vi "Inspect VI.vi"(7 "Inspector Config":T1, 8 "error in (no error)":errorcluster, 11 "VI Path":path=path "C:/dev/SoL/sol-word-search/Scorer (2024Q1)/Scorer/Naughty VI Test.vi") -> (0 "error out":errorcluster, 2 "Issues":string[](array[string]), 3 "Result":bool)   [LabVIEW 2020, in "SoL Inspector.lvlib"]
uses:
  SoL Inspector.lvlib
  Inspector Config.ctl
  Inspection.ctl
  <vilib>/Utility/traverseref.llb/TRef TravTarget.ctl
  <vilib>/Utility/traverseref.llb/VI Scripting - Traverse.lvlib
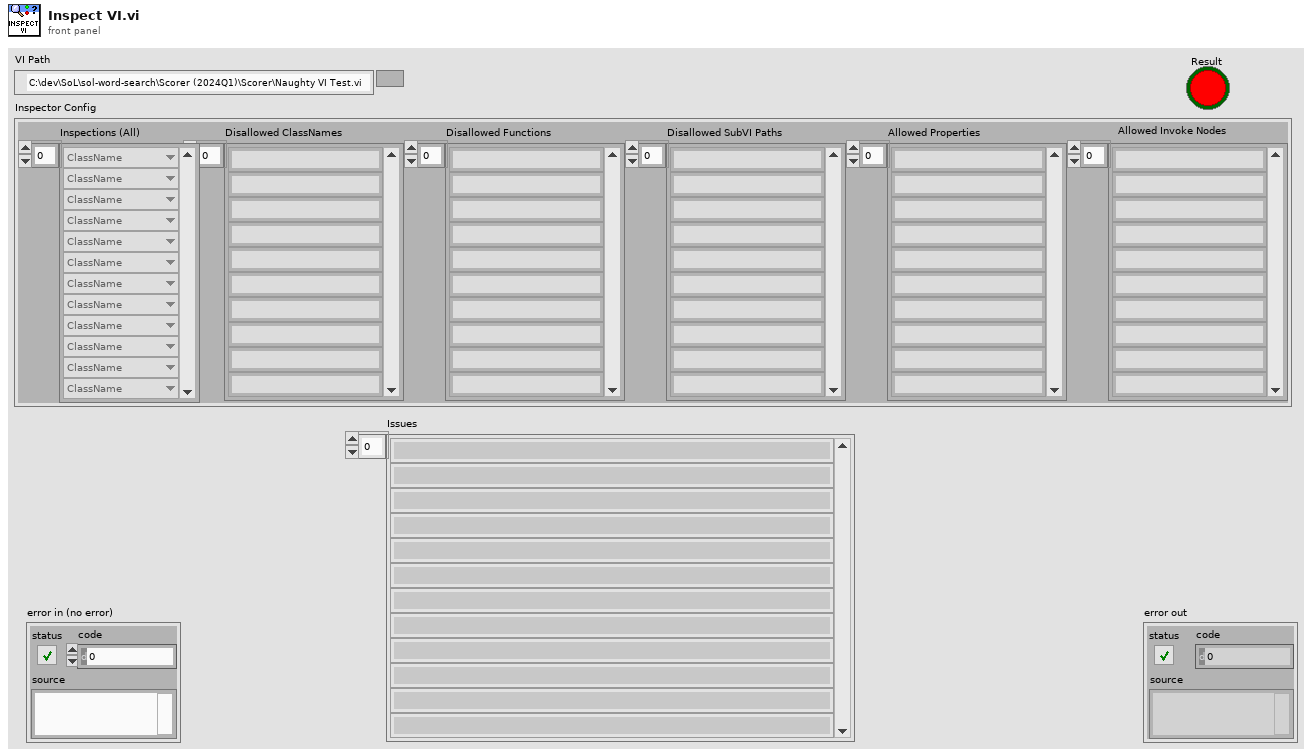
[diagram p1: front panel]
types:
  T1 = typedef "SoL Inspector.lvlib/Inspector Config.ctl" = cluster{"Inspections (All)":T2[], "Disallowed ClassNames":string[], "Disallowed Functions":string[], "Disallowed SubVI Paths":string[], "Allowed Properties":string[], "Allowed Invoke Nodes":string[]}
  T2 = typedef "SoL Inspector.lvlib/Inspection.ctl" = enum16{"ClassName", "Functions", "CallLibrary", "SubVIs", "FileIO", "Invoke Nodes", "Properties", "Growable Functions"}
  T3 = typedef "TRef TravTarget.ctl" = enum16{"FP", "BD", "Other"}
  T4 = typedef "ASPM_UniqueIDStringDatanameShortnameLongname.ctl" = cluster{"Unique ID string":string, "Data name":string, "Short name (localized)":string, "Long name (localized)":string}
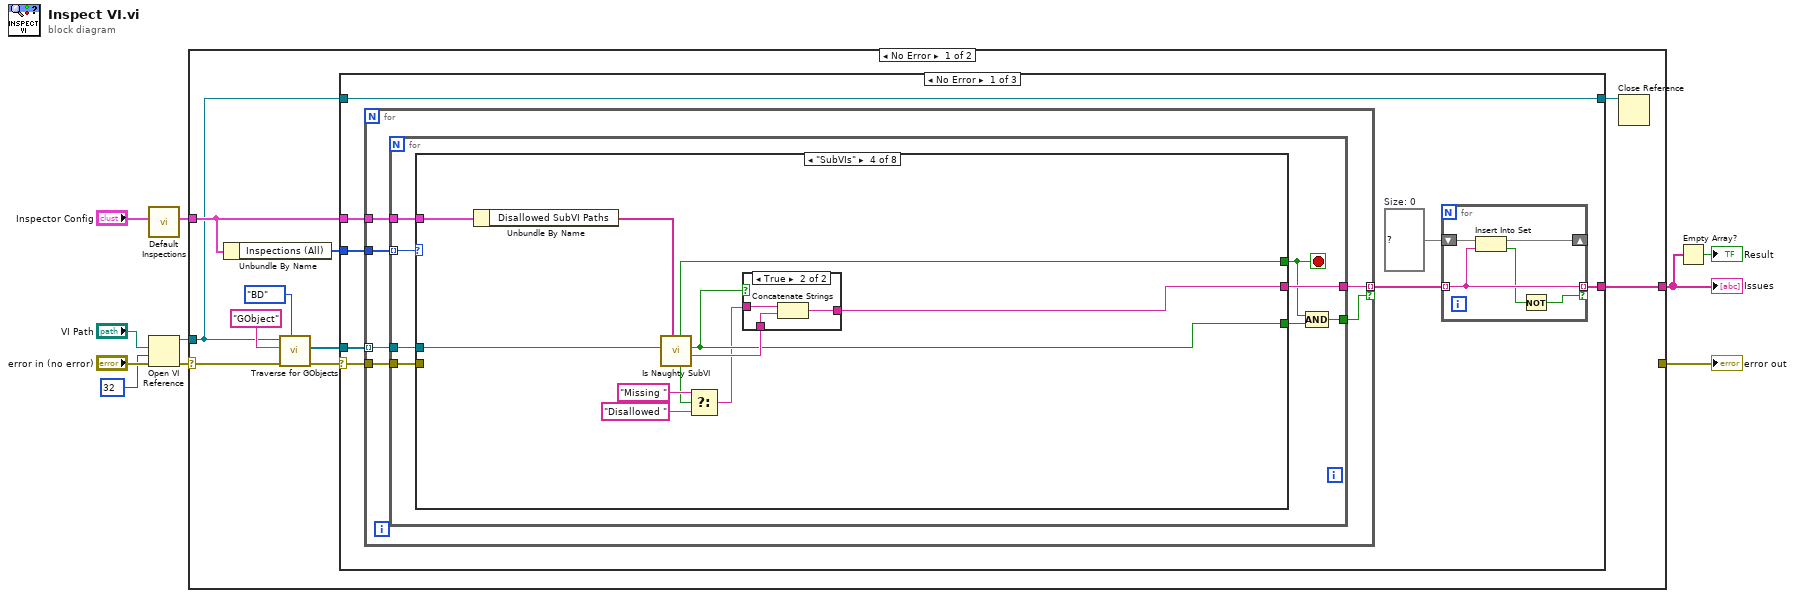
[diagram p0: block diagram]
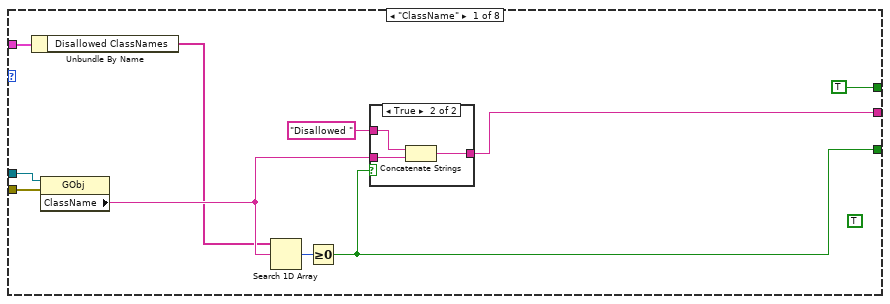
[diagram p2: hidden frame]
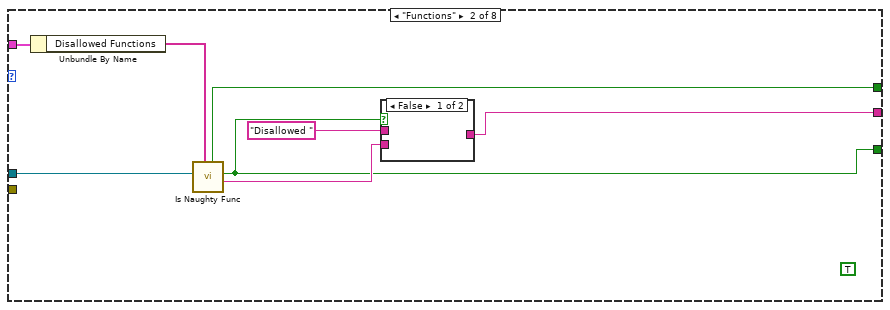
[diagram p4: hidden frame]
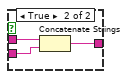
[diagram p5: hidden frame]
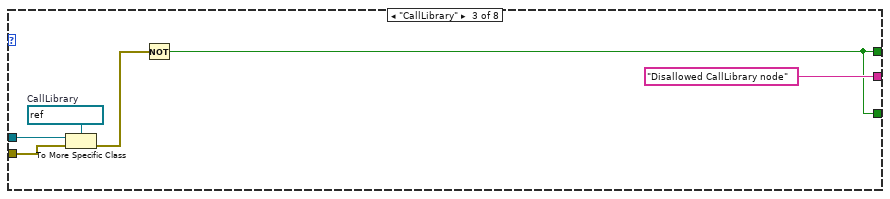
[diagram p6: hidden frame]
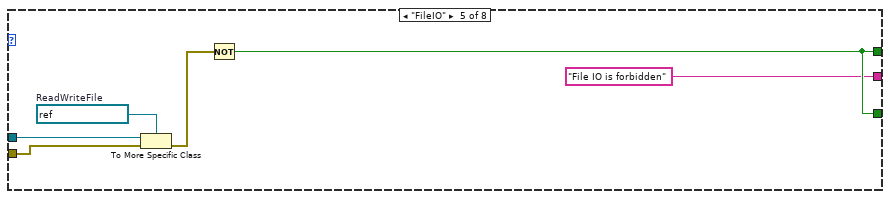
[diagram p8: hidden frame]
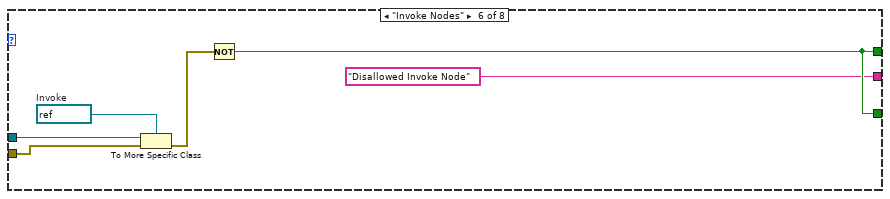
[diagram p9: hidden frame]
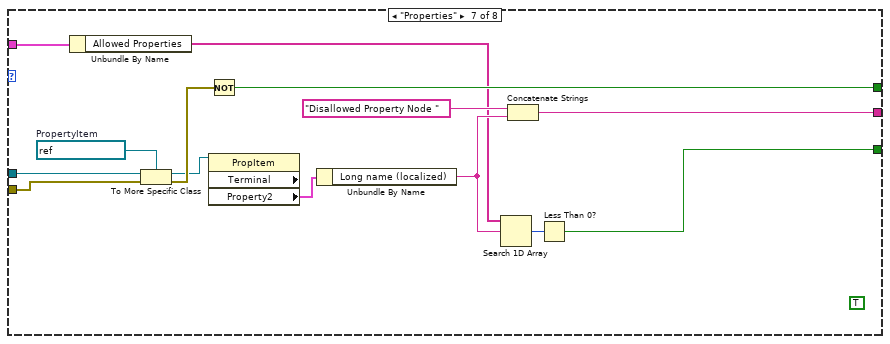
[diagram p10: hidden frame]
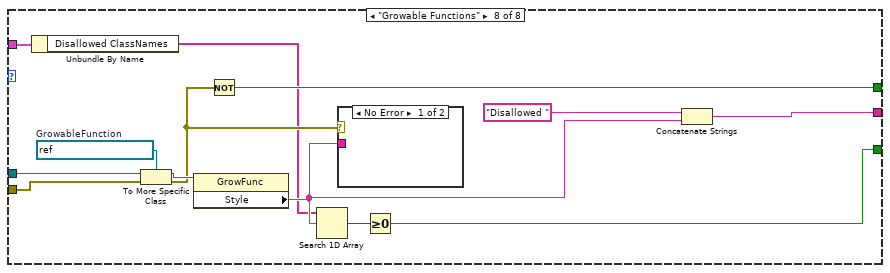
[diagram p11: hidden frame]
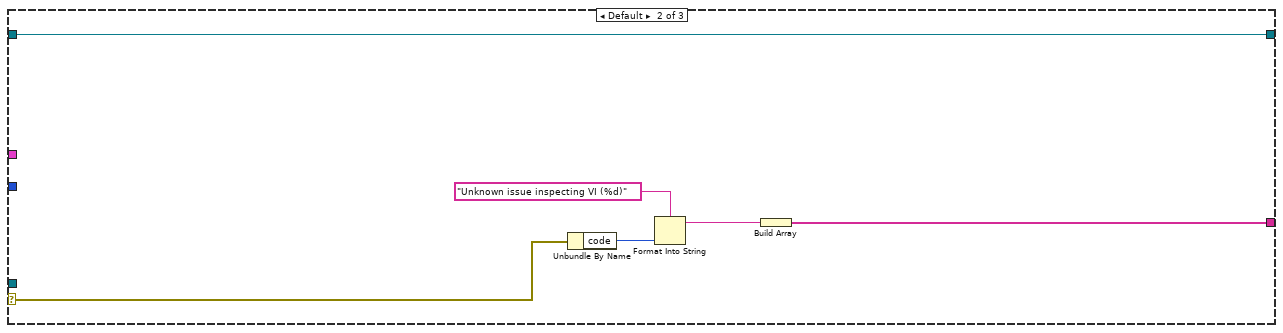
[diagram p13: hidden frame]
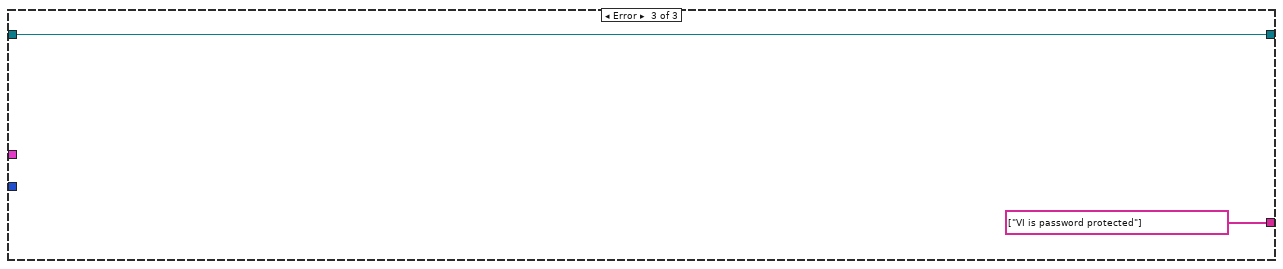
[diagram p14: hidden frame]
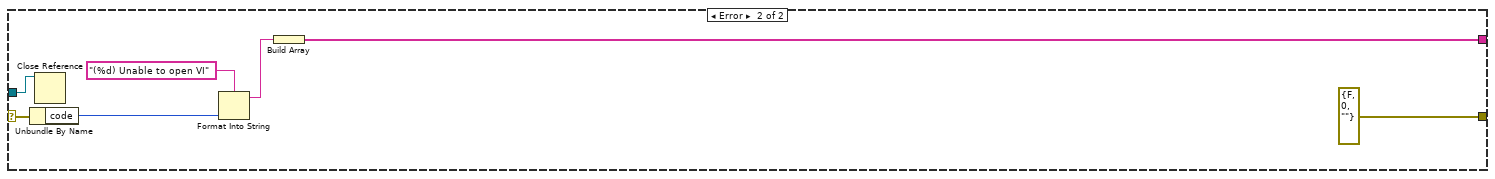
[diagram p15: hidden frame]
diagram:
  n1 = call "Default Inspections.vi"("Inspector Config in"="Inspector Config") -> ("Inspector Config"=w3:T1)  [unwired: 10 in]
  n2 = Open VI Reference(vi path="VI Path", options=32, error in (no error)="error in (no error)") -> (vi reference=w6:refnum<vi>, error out=w7:errorcluster)  [unwired: 3 in]
  n3 = case shown="No Error" w7 {
    selector: w7 -> [w20 w143]
    tunnel: w6 -> [w12 w144]
    tunnel: [w15 w139] -> w2
    tunnel: [_ errorcluster {"status"=FALSE, "code"=0, "source"=""} ("error constant")] -> w5
    tunnel: w3 -> [w13 _]
    frame No Error {
      n4 = Unbundle By Name(w13) -> ("Inspections (All)"=w14:T2[])
      n5 = call <vilib>:"Traverse for GObjects.vi"("Traverse Target"=TRef_TravTarget."BD", "error in (no error)"=w20, "Class Name"="GObject", "VI Refnum"=w12) -> ("error out"=w16:errorcluster, "References"=w17:refnum<vi>[])  [unwired: 4 in, 2 out]
      n6 = case shown="No Error" w16 {
        selector: w16 -> [w27 w132 _]
        tunnel: w17 -> [w28 _ _]
        tunnel: [w24 w133 string[] ["VI is password protected"]] -> w15
        tunnel: w14 -> [w23 _ _]
        tunnel: w13 -> [w22 _ _]
        tunnel: w12 -> [w21 w131 w137]
        tunnel: [w21 w131 w137] -> w11
        frame No Error {
          w25 = set{string} {}  # Size: 0
          n7 = for {
            tunnel: w28 -> [w34] mode=indexing
            tunnel: w27 -> [w33]
            tunnel: [w32] -> w26 mode=indexing if=w31
            tunnel: w23 -> [w30]
            tunnel: w22 -> [w29]
            n8 = for {
              tunnel: w34 -> [w42]
              tunnel: w33 -> [w41]
              tunnel: [w40] -> w32
              tunnel: [w36] -> w31
              tunnel: w30 -> [w38] mode=indexing
              tunnel: w29 -> [w37]
              stop <- w35 stop-if-true
              n9 = case shown="\"SubVIs\"" w38 {
                tunnel: [TRUE w58 w67 w83 w88 w94 w107 w119] -> w35
                tunnel: w42 -> [w50 w63 w72 w79 w92 w98 w112 w125]
                tunnel: w41 -> [w51 _ w71 _ w91 w97 w111 w124]
                tunnel: [w45 w60 "Disallowed CallLibrary node" w81 "File IO is forbidden" "Disallowed Invoke Node" w103 w116] -> w40
                tunnel: [w48 w59 w67 w80 w88 w94 w104 w118] -> w39
                tunnel: w37 -> [w44 w57 _ w74 _ _ w100 w114]
                frame "ClassName" {
                  (unwired) TRUE
                  n10 = Unbundle By Name(w44) -> ("Disallowed ClassNames"=w43:string[])
                  n11 = property class="GObj"(reference=w50, error in=w51) -> ("ClassName"=w46:string)  [unwired: 2 out]
                  n12 = Search 1D Array(1D array=w43, element=w46) -> (index of element=w49:i32)  [unwired: 1 in]
                  n13 = Greater Or Equal To 0?(x=w49) -> (x >= 0?=w48:bool)
                  n14 = case shown="True" w48 {
                    tunnel: "Disallowed " -> [_ w55]
                    tunnel: w46 -> [_ w54]
                    tunnel: [_ w53] -> w45
                    frame False {
                    }
                    frame True {
                      n15 = Concatenate Strings(w55, w54) -> (w53:string)
                    }
                  }
                }
                frame "Functions" {
                  (unwired) TRUE
                  n16 = Unbundle By Name(w57) -> ("Disallowed Functions"=w56:string[])
                  n17 = call "Is Naughty Func.vi"("Disallowed Functions"=w56, "GObj Refnum"=w63) -> ("Function"=w61:string, "Naughty Function"=w59:bool, "Is Func"=w58:bool)  [unwired: 7 in]
                  n18 = case shown="False" w59 {
                    tunnel: "Disallowed " -> [_ w66]
                    tunnel: w61 -> [_ w65]
                    tunnel: [_ w64] -> w60
                    frame False {
                    }
                    frame True {
                      n19 = Concatenate Strings(w66, w65) -> (w64:string)
                    }
                  }
                }
                frame "CallLibrary" {
                  w70 = refnum<vi> refnum  # CallLibrary
                  n20 = To More Specific Class(target class=w70, reference=w72, error in=w71) -> (error out=w69:errorcluster)  [unwired: 1 out]
                  n21 = Not(x=w69) -> (.not. x?=w67:bool)
                }
                frame "SubVIs" {
                  n22 = Unbundle By Name(w74) -> ("Disallowed SubVI Paths"=w73:string[])
                  n23 = call "Is Naughty SubVI.vi"("Disallowed SubVI Paths"=w73, "GObj Refnum"=w79) -> ("SubVI"=w82:string, "Naughty SubVI"=w80:bool, "Missing SubVI"=w75:bool, "Is SubVI"=w83:bool)  [unwired: 5 in, 1 out]
                  n24 = Select(t="Missing ", s=w75, f="Disallowed ") -> (s? t:f=w77:string)
                  n25 = case shown="True" w80 {
                    tunnel: w77 -> [_ w86]
                    tunnel: w82 -> [_ w85]
                    tunnel: [_ w84] -> w81
                    frame False {
                    }
                    frame True {
                      n26 = Concatenate Strings(w86, w85) -> (w84:string)
                    }
                  }
                }
                frame "FileIO" {
                  w90 = refnum<vi> refnum  # ReadWriteFile
                  n27 = To More Specific Class(target class=w90, reference=w92, error in=w91) -> (error out=w89:errorcluster)  [unwired: 1 out]
                  n28 = Not(x=w89) -> (.not. x?=w88:bool)
                }
                frame "Invoke Nodes" {
                  w96 = refnum<vi> refnum  # Invoke
                  n29 = To More Specific Class(target class=w96, reference=w98, error in=w97) -> (error out=w95:errorcluster)  [unwired: 1 out]
                  n30 = Not(x=w95) -> (.not. x?=w94:bool)
                }
                frame "Properties" {
                  (unwired) TRUE
                  w110 = refnum<vi> refnum  # PropertyItem
                  n31 = Unbundle By Name(w100) -> ("Allowed Properties"=w99:string[])
                  n32 = To More Specific Class(target class=w110, reference=w112, error in=w111) -> (specific class reference=w101:refnum<vi>, error out=w109:errorcluster)
                  n33 = Not(x=w109) -> (.not. x?=w107:bool)
                  n34 = property class="PropItem" props=["Terminal", "Property2"](reference=w101) -> ("Property2"=w106:T4)  [unwired: 1 in, 3 out]
                  n35 = Unbundle By Name(w106) -> ("Long name (localized)"=w102:string)
                  n36 = Search 1D Array(1D array=w99, element=w102) -> (index of element=w105:i32)  [unwired: 1 in]
                  n37 = Concatenate Strings("Disallowed Property Node ", w102) -> (w103:string)
                  n38 = Less Than 0?(x=w105) -> (x < 0?=w104:bool)
                }
                frame "Growable Functions" {
                  w123 = refnum<vi> refnum  # GrowableFunction
                  n39 = Unbundle By Name(w114) -> ("Disallowed ClassNames"=w113:string[])
                  n40 = To More Specific Class(target class=w123, reference=w125, error in=w124) -> (specific class reference=w121:refnum<vi>, error out=w117:errorcluster)
                  n41 = property class="GrowFunc"(reference=w121) -> ("Style"=w115:string)  [unwired: 1 in, 2 out]
                  n42 = Not(x=w117) -> (.not. x?=w119:bool)
                  n43 = Search 1D Array(1D array=w113, element=w115) -> (index of element=w120:i32)  [unwired: 1 in]
                  n44 = case shown="No Error" w117 {
                    tunnel: w115 -> [_ _]
                    frame No Error {
                    }
                    frame Error {
                    }
                  }
                  n45 = Greater Or Equal To 0?(x=w120) -> (x >= 0?=w118:bool)
                  n46 = Concatenate Strings("Disallowed ", w115) -> (w116:string)
                }
              }
              n47 = Compound Arithmetic op=AND(w35, w39) -> (w36:bool)
            }
          }
          n48 = for {
            tunnel: w26 -> [w128] mode=indexing
            shift-right: [w129] -> _
            shift-left: w25 -> [w130]
            tunnel: [w128] -> w24 mode=indexing if=w126
            n49 = Insert Into Set(10:w128, 11:w130) -> (2:w127:bool, 3:w129:set{string})
            n50 = Not(x=w127) -> (.not. x?=w126:bool)
          }
        }
        frame Default {
          n51 = Unbundle By Name(w132) -> ("code"=w135:i32)
          n52 = Format Into String(format string="Unknown issue inspecting VI (%d)", w135) -> (resulting string=w134:string)  [unwired: 2 in, 1 out]
          n53 = Build Array(w134) -> (w133:string[])
        }
        frame Error {
        }
      }
      n54 = Close Reference(reference=w11) -> ()  [unwired: 1 in, 1 out]
    }
    frame Error {
      n55 = Unbundle By Name(w143) -> ("code"=w142:i32)
      n56 = Close Reference(reference=w144) -> ()  [unwired: 1 in, 1 out]
      n57 = Format Into String(format string="(%d) Unable to open VI", w142) -> (resulting string=w140:string)  [unwired: 2 in, 1 out]
      n58 = Build Array(w140) -> (w139:string[])
    }
  }
  "error out" <- w5
  "Issues" <- w2
  n59 = Empty Array?(array=w2) -> (empty?=→"Result":bool)
